vi "W9EO82,FBO8PP_21.vi"(10 "Slide":i32, 11 "Numeric in":dbl) -> (2 "String":string, 3 "Numeric out":dbl)   [LabVIEW 2021]
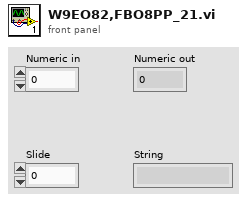
[diagram p1: front panel]
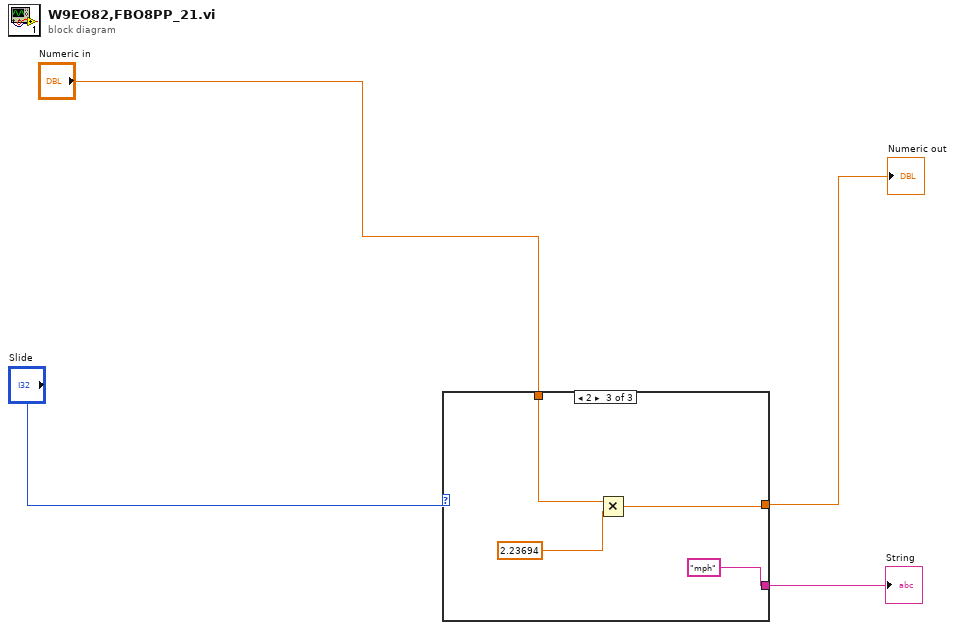
[diagram p0: block diagram]
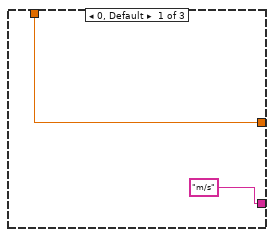
[diagram p2: hidden frame]
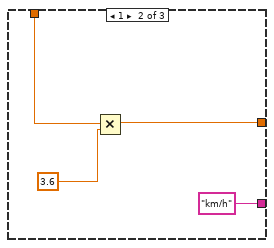
[diagram p3: hidden frame]
diagram:
  n1 = case shown="2" "Slide" {
    tunnel: "Numeric in" -> [w6 w9 w13]
    tunnel: [w6 w10 w12] -> w3
    tunnel: ["m/s" "km/h" "mph"] -> w4
    frame 0, Default {
    }
    frame 1 {
      n2 = Multiply(x=w9, y=3.6) -> (x*y=w10:dbl)
    }
    frame 2 {
      n3 = Multiply(x=w13, y=2.23694) -> (x*y=w12:dbl)
    }
  }
  "String" <- w4
  "Numeric out" <- w3
